vi "TSM SSC DAQmx Write (Digital Bool 1Samp) Per-Site Per-Pin.vi"(0 "DAQ TSM in":T1, 7 "Per-Site Per-Pin Waveforms in":bool[][](array[boolean]), 11 "error in":errorcluster) -> (4 "DAQ TSM Out":T1, 15 "error out":errorcluster)   [LabVIEW 2020]
doc: "Writes one or more waveforms to a task that contains one or more analog output channels. The waveform data should be in the same order as SSC."
uses:
  Pin Map/TSM DAQmx Multi-Task.ctl
  <vilib>/NI_TestStand_SemiconductorModule/NI_TestStand_Semiconductor_Module.lvlibp/PinMap/PinQueryContext/MultiplePinMultipleSessionQueryContext/MultiplePinMultipleSessionQueryContext.lvclass
  Pin Map/SSC DAQmx.ctl
  7682f338-adbd-462d-a0ce-32ef4d99d3be.vi
  <vilib>/DAQmx/write.llb/DAQmx Write (Digital 1D Bool NChan 1Samp 1Line).vi
  <vilib>/DAQmx/miscellaneous.llb/DAQmx Fill In Error Info.vi
  <resource>/objmgr/daqmx.rc
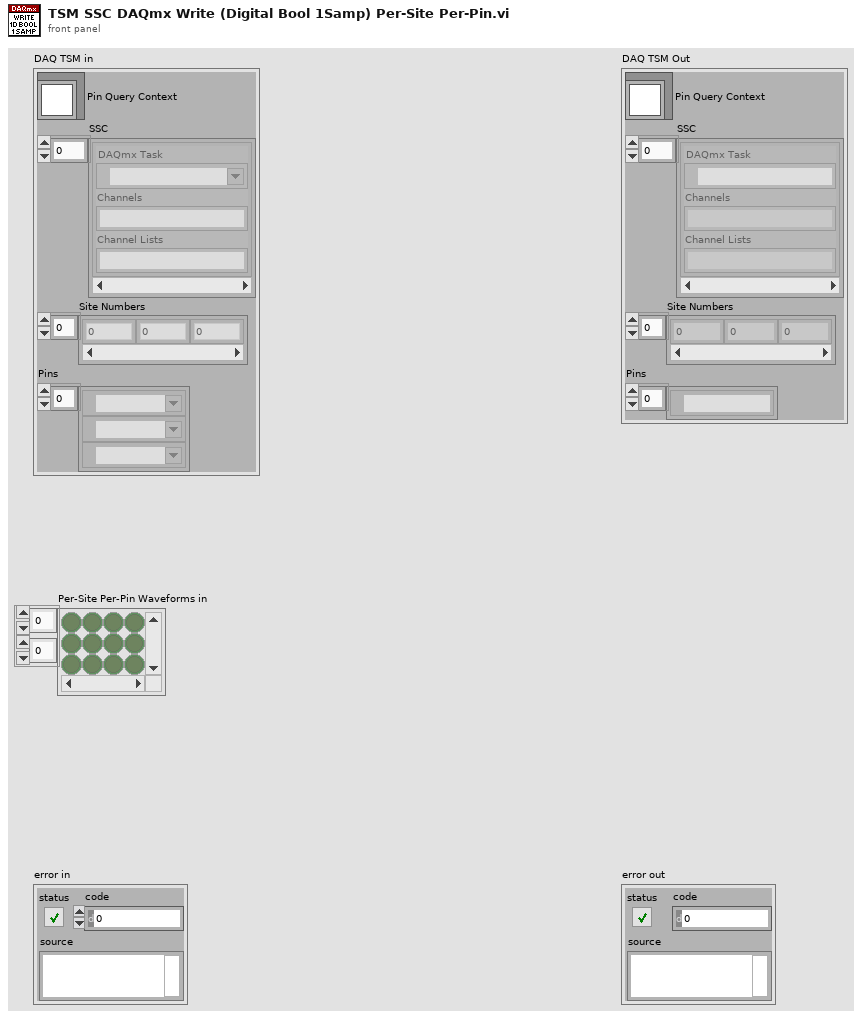
[diagram p1: front panel]
types:
  T1 = typedef "TSM DAQmx Multi-Task.ctl" = cluster{"Pin Query Context":refnum<class "MultiplePinMultipleSessionQueryContext.lvclass">, "SSC":T2[], "Site Numbers":i32[], "Pins":tag[]}
  T2 = typedef "SSC DAQmx.ctl" = cluster{"DAQmx Task ":refnum<k21>, "Channels":string, "Channel Lists":string}
  T3 = typedef "Digital 2D Location.ctl" = cluster{"Row":i32, "Col":i32}
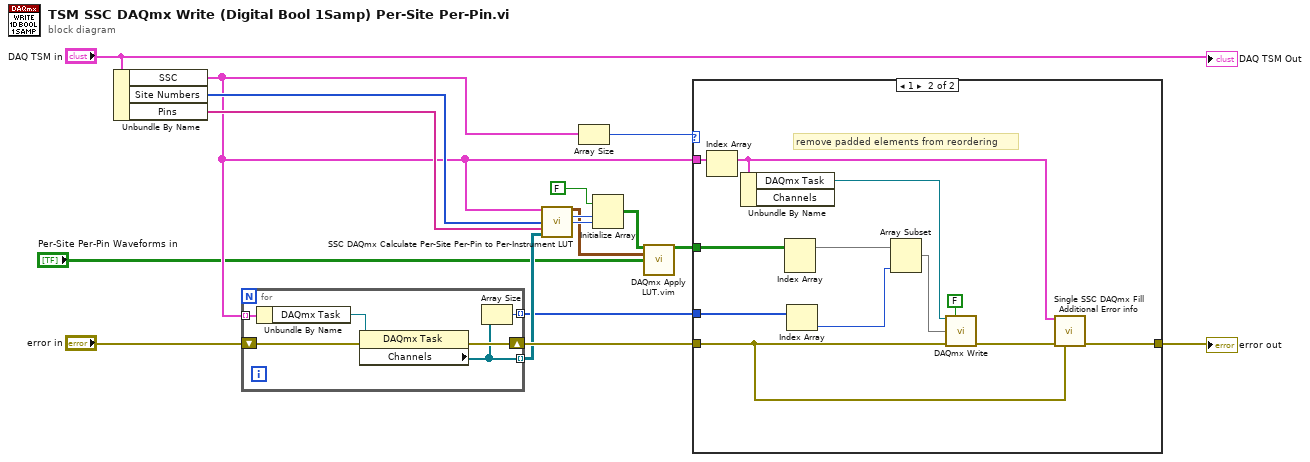
[diagram p0: block diagram]
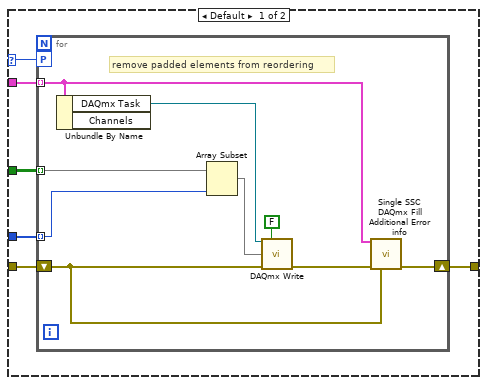
[diagram p2: hidden frame]
diagram:
  n1 = Unbundle By Name("DAQ TSM in") -> ("SSC"=w7:T2[], "Site Numbers"=w14:i32[], "Pins"=w13:tag[])
  n2 = for {
    shift-right: [w22] -> w8
    shift-left: "error in" -> [w23]
    tunnel: w7 -> [w21] mode=indexing
    tunnel: [w19] -> w6 mode=indexing
    tunnel: [w18] -> w5 mode=indexing
    n3 = Unbundle By Name(w21) -> ("DAQmx Task"=w20:refnum<k21>)
    n4 = property class="DAQmx Task"(reference=w20, error in=w23) -> (error out=w22:errorcluster, "Channels"=w19:refnum<k21>[])  [unwired: 1 out]
    n5 = Array Size(array=w19) -> (size(s)=w18:i32)
  }
  n6 = call "SSC DAQmx Calculate Per-Site Per-Pin to Per-Instrument LUT.vi"("DAQmx SSC in"=w7, "Sites"=w14, "Pins"=w13, "AO Channels"=w6) -> ("Per-Site Per-Pin to Per-Task LUT"=w10:T3[][], "Task Count"=w12:i32, "Max Channels in a Task"=w11:i32)  [unwired: 9 in]
  n7 = Array Size(array=w7) -> (size(s)=w9:i32)
  n8 = Initialize Array(FALSE, w12, w11) -> (w1:bool[][])
  n9 = call "DAQmx Apply LUT.vim"("Initialized Array"=w1, "LUT"=w10, "Results to Apply LUT to"="Per-Site Per-Pin Waveforms in") -> ("Array Out"=w4:bool[][])  [unwired: 12 in]
  n10 = case shown="1" w9 {
    selector: w9 -> [w27 _]
    tunnel: [w29 w50] -> w15
    tunnel: w8 -> [w28 w49]
    tunnel: w7 -> [w26 w48]
    tunnel: w4 -> [w25 w47]
    tunnel: w5 -> [w24 w46]
    frame Default {
      n11 = for {
        tunnel: w26 -> [w35] mode=indexing
        workers-P: w27 -> [_]
        shift-right: [w38] -> w29
        shift-left: w28 -> [w37]
        tunnel: w25 -> [w33] mode=indexing
        tunnel: w24 -> [w32] mode=indexing
        # "remove padded elements from reordering"
        n12 = Unbundle By Name(w35) -> ("DAQmx Task"=w34:refnum<k21>)  [unwired: 1 out]
        n13 = Array Subset(array=w33, length=w32) -> (w31:bool[])  [unwired: 1 in]
        n14 = call-poly <vilib>:"DAQmx Write.vi"("task/channels in"=w34, "auto start"=FALSE, "data"=w31, "error in"=w37) -> ("error out"=w36:errorcluster)  [unwired: 9 in, 2 out]
        n15 = call "Single SSC DAQmx Fill Additional Error info.vi"("DAQmx SSC in"=w35, "error in"=w36, "previous error in"=w37) -> ("error out"=w38:errorcluster)  [unwired: 12 in]
      }
    }
    frame 1 {
      # "remove padded elements from reordering"
      n16 = Index Array(array=w48) -> (element=w43:T2)  [unwired: 1 in]
      n17 = Unbundle By Name(w43) -> ("DAQmx Task"=w44:refnum<k21>)  [unwired: 1 out]
      n18 = Index Array(array=w47) -> (element=w41:bool[])  [unwired: 2 in]
      n19 = Index Array(array=w46) -> (element=w42:i32)  [unwired: 1 in]
      n20 = Array Subset(array=w41, length=w42) -> (w40:bool[])  [unwired: 1 in]
      n21 = call-poly <vilib>:"DAQmx Write.vi"("task/channels in"=w44, "auto start"=FALSE, "data"=w40, "error in"=w49) -> ("error out"=w45:errorcluster)  [unwired: 9 in, 2 out]
      n22 = call "Single SSC DAQmx Fill Additional Error info.vi"("DAQmx SSC in"=w43, "error in"=w45, "previous error in"=w49) -> ("error out"=w50:errorcluster)  [unwired: 12 in]
    }
  }
  "error out" <- w15
  "DAQ TSM Out" <- "DAQ TSM in"
